vi "Input1.vi"(7 "Drag":dbl, 8 "Remapped Frame Properties":T1, 10 "Signal in":dbl) -> ()   [LabVIEW 2019]
uses:
  <userlib>/HapticSTM/HapticSTM.lvlib
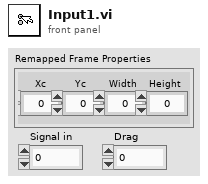
[diagram p1: front panel]
types:
  T1 = cluster{"Xc":dbl, "Yc":dbl, "Width":dbl, "Height":dbl}
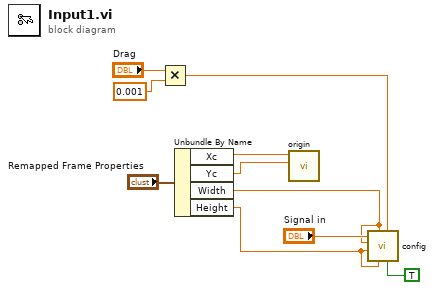
[diagram p0: block diagram]
diagram:
  n1 = Multiply(x="Drag", y=0.001) -> (x*y=w8:dbl)
  n2 = Unbundle By Name("Remapped Frame Properties") -> ("Xc"=w3:dbl, "Yc"=w4:dbl, "Width"=w2:dbl, "Height"=w1:dbl)
  n3 = call <userlib>:"origin.vi"("zorg"=w4, "xorg"=w3) -> ()  [unwired: 10 in]
  n4 = call <userlib>:"config.vi"("feedback"=TRUE, "dragc"=w8, "sizeofimgz"=w1, "sizeofimgx"=w2, "scopez"=w1, "scopex"=w2, "ypos"="Signal in") -> ()  [unwired: 5 in]
